vi "CreateSourceNode.vi"(7 "DOM Document":refnum<k20>, 8 "Error In":errorcluster, 11 "Source Configuration":T1={"Enabled?"=TRUE, "Function"=enum."Voltage", "Level (V or A)"=1.0, "Autorange Enabled?"=FALSE, "High Limit (V or A)"=0.0, "Low Limit (V or A)"=0.0}) -> (0 "Error Out":errorcluster, 3 "Source Node":refnum<k20>)   [LabVIEW 2013]
uses:
  SourceConfiguration.ctl
  SourceFunction.ctl
  libs/LV-Utilities/LV-Utilities.lvlib
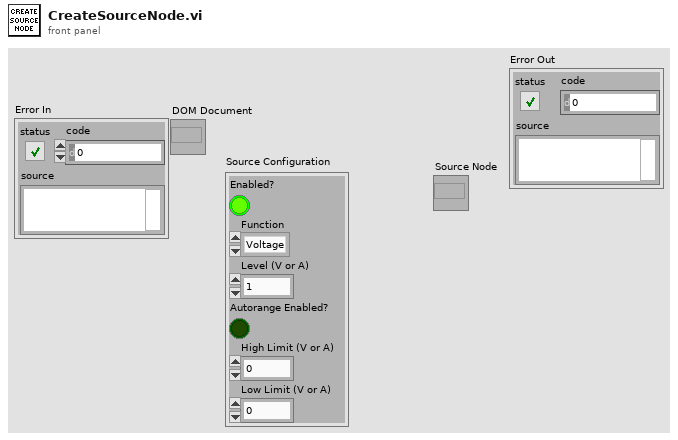
[diagram p1: front panel]
types:
  T1 = typedef "SourceConfiguration.ctl" = cluster{"Enabled?":bool, "Function":T2, "Level (V or A)":dbl, "Autorange Enabled?":bool, "High Limit (V or A)":dbl, "Low Limit (V or A)":dbl}
  T2 = typedef "SourceFunction.ctl" = enum16{"Voltage", "Current"}
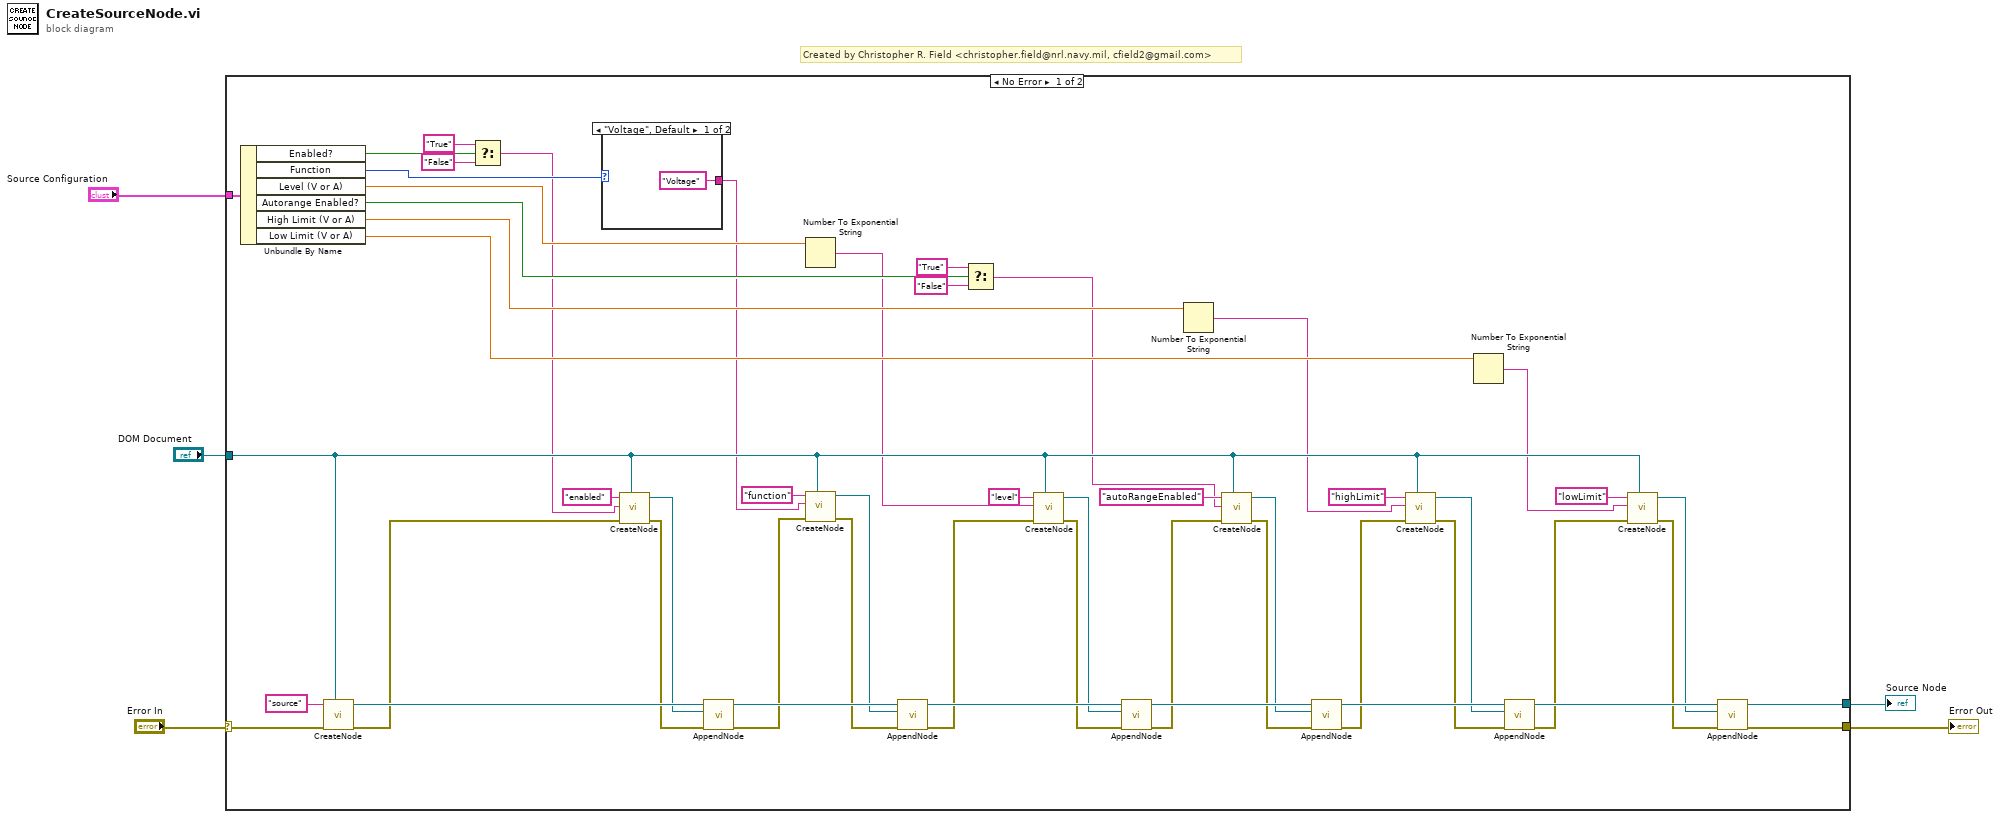
[diagram p0: block diagram]
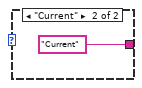
[diagram p2: hidden frame]
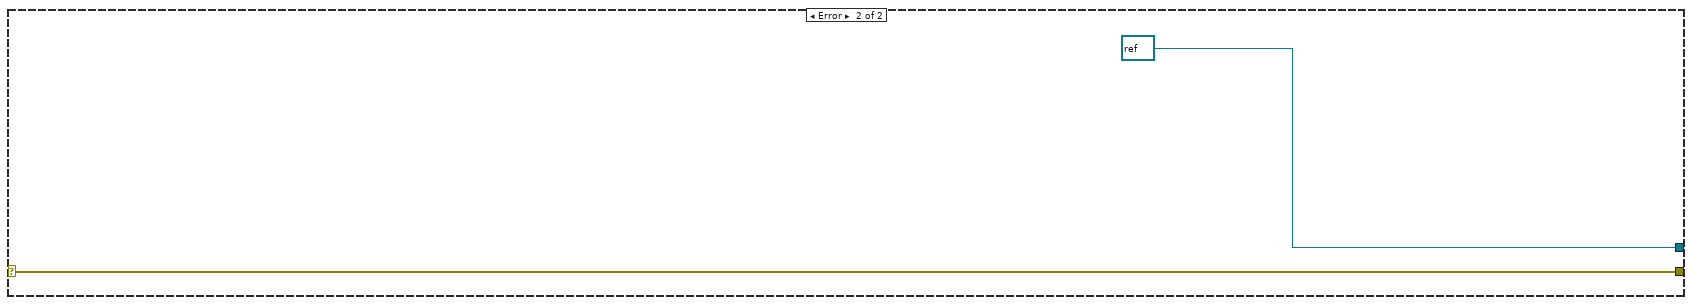
[diagram p3: hidden frame]
diagram:
  # "Created by Christopher R. Field <christopher.field@nrl.navy.mil, cfield2@gmail.com>"
  n1 = case shown="No Error" "Error In" {
    selector: "Error In" -> [w45 w61]
    tunnel: "DOM Document" -> [w29 _]
    tunnel: [w32 refnum<k20> refnum ("Wirings Node 2")] -> w3
    tunnel: [w31 w61] -> w2
    tunnel: "Source Configuration" -> [w57 _]
    frame No Error {
      n2 = Unbundle By Name(w57) -> ("Enabled?"=w56:bool, "Function"=w53:T2, "Level (V or A)"=w52:dbl, "Autorange Enabled?"=w49:bool, "High Limit (V or A)"=w48:dbl, "Low Limit (V or A)"=w47:dbl)
      n3 = call "CreateNode.vi"("DOM Document"=w29, "Error In"=w45, "Tag Name"="source") -> ("Error out"=w30:errorcluster, "Node"=w38:refnum<k20>)  [unwired: 7 in]
      n4 = Select(t="True", s=w56, f="False") -> (s? t:f=w11:string)
      n5 = case shown="\"Voltage\", Default" w53 {
        tunnel: ["Voltage" "Current"] -> w10
        frame "Voltage", Default {
        }
        frame "Current" {
        }
      }
      n6 = call "CreateNode.vi"("DOM Document"=w29, "Error In"=w30, "Text"=w11, "Tag Name"="enabled") -> ("Error out"=w28:errorcluster, "Node"=w12:refnum<k20>)  [unwired: 6 in]
      n7 = call "AppendNode.vi"("Error In"=w28, "Child Node"=w12, "Parent Node In"=w38) -> ("Error Out"=w27:errorcluster, "Parent Node Out"=w37:refnum<k20>)  [unwired: 7 in]
      n8 = Number To Exponential String(number=w52) -> (E-format string=w9:string)  [unwired: 3 in]
      n9 = call "CreateNode.vi"("DOM Document"=w29, "Error In"=w27, "Text"=w10, "Tag Name"="function") -> ("Error out"=w26:errorcluster, "Node"=w13:refnum<k20>)  [unwired: 6 in]
      n10 = call "AppendNode.vi"("Error In"=w26, "Child Node"=w13, "Parent Node In"=w37) -> ("Error Out"=w25:errorcluster, "Parent Node Out"=w36:refnum<k20>)  [unwired: 7 in]
      n11 = Select(t="True", s=w49, f="False") -> (s? t:f=w8:string)
      n12 = call "CreateNode.vi"("DOM Document"=w29, "Error In"=w25, "Text"=w9, "Tag Name"="level" ("Text")) -> ("Error out"=w24:errorcluster, "Node"=w14:refnum<k20>)  [unwired: 6 in]
      n13 = call "AppendNode.vi"("Error In"=w24, "Child Node"=w14, "Parent Node In"=w36) -> ("Error Out"=w23:errorcluster, "Parent Node Out"=w35:refnum<k20>)  [unwired: 7 in]
      n14 = Number To Exponential String(number=w48) -> (E-format string=w7:string)  [unwired: 3 in]
      n15 = call "CreateNode.vi"("DOM Document"=w29, "Error In"=w23, "Text"=w8, "Tag Name"="autoRangeEnabled") -> ("Error out"=w22:errorcluster, "Node"=w15:refnum<k20>)  [unwired: 6 in]
      n16 = call "AppendNode.vi"("Error In"=w22, "Child Node"=w15, "Parent Node In"=w35) -> ("Error Out"=w21:errorcluster, "Parent Node Out"=w34:refnum<k20>)  [unwired: 7 in]
      n17 = call "CreateNode.vi"("DOM Document"=w29, "Error In"=w21, "Text"=w7, "Tag Name"="highLimit") -> ("Error out"=w20:errorcluster, "Node"=w16:refnum<k20>)  [unwired: 6 in]
      n18 = Number To Exponential String(number=w47) -> (E-format string=w6:string)  [unwired: 3 in]
      n19 = call "AppendNode.vi"("Error In"=w20, "Child Node"=w16, "Parent Node In"=w34) -> ("Error Out"=w19:errorcluster, "Parent Node Out"=w33:refnum<k20>)  [unwired: 7 in]
      n20 = call "CreateNode.vi"("DOM Document"=w29, "Error In"=w19, "Text"=w6, "Tag Name"="lowLimit") -> ("Error out"=w18:errorcluster, "Node"=w17:refnum<k20>)  [unwired: 6 in]
      n21 = call "AppendNode.vi"("Error In"=w18, "Child Node"=w17, "Parent Node In"=w33) -> ("Error Out"=w31:errorcluster, "Parent Node Out"=w32:refnum<k20>)  [unwired: 7 in]
    }
    frame Error {
    }
  }
  "Source Node" <- w3
  "Error Out" <- w2
